vi "test2-DifferentChainNodesProcessDifferentAllowedMessages.vi"(8 "error in (no error)":errorcluster, 11 "TestCase in":refnum<class "testcase-CSMChainMode.lvclass">) -> (0 "error out":errorcluster, 3 "TestCase out":refnum<class "testcase-CSMChainMode.lvclass">)   [LabVIEW 2017, in "testcase-CSMChainMode.lvclass"]
uses:
  testcase-CSMChainMode.lvclass
  <vilib>/addons/_JKI Toolkits/VI Tester/TestCase.llb/TestCase.lvclass
  src/user.lib/_NEVSTOP/Communicable State Machine(CSM)/Communicable State Machine.lvlib
  C:/Program Files (x86)/National Instruments/LabVIEW 2017/vi.lib/addons/_JKI Toolkits/VI Tester/TestCase.llb/TestCase.lvclass
panel:
  out "LoopCount":i32
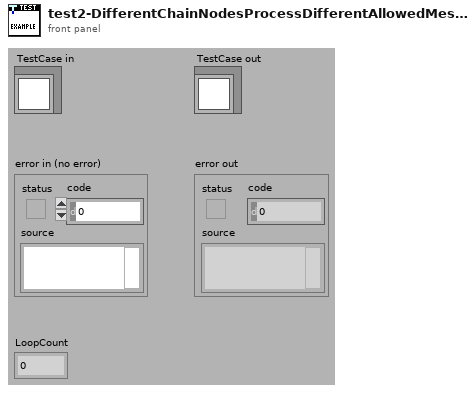
[diagram p1: front panel]
types:
  T1 = cluster{"Allowed":string, "Not Allowed":string[]}[]
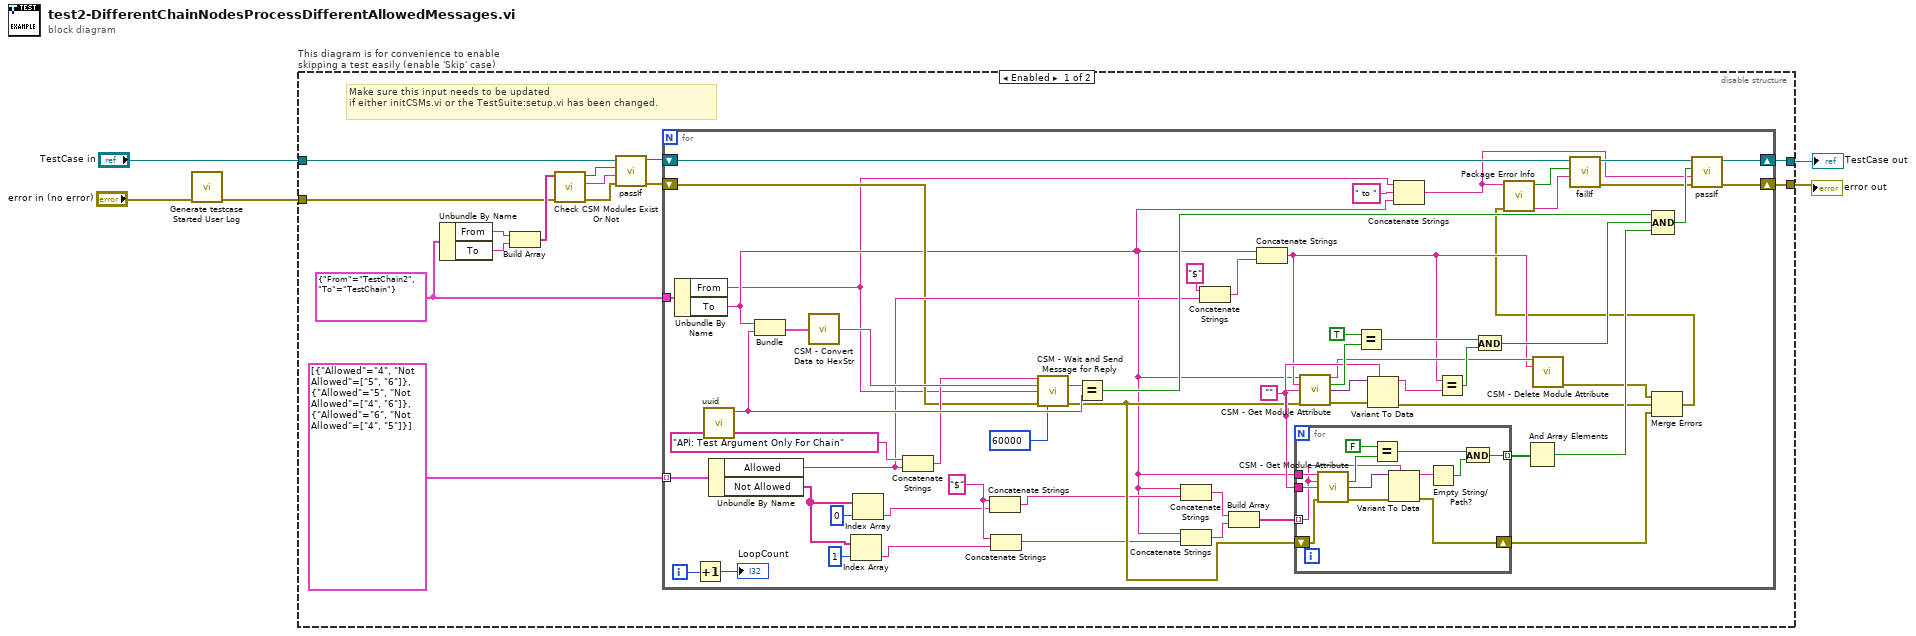
[diagram p0: block diagram]
diagram:
  n1 = call "Generate testcase Started User Log.vi"("Error In"="error in (no error)") -> ("error out"=w1:errorcluster)  [unwired: 10 in]
  n2 = disable-structure "This diagram is for convenience to enable skipping a test easily (enable 'Skip' case)" shown="Enabled" {
    disable-tunnel: "TestCase in" -> [w10 w93]
    disable-tunnel: [w19 w91] -> w2
    disable-tunnel: [w18 w92] -> w4
    disable-tunnel: w1 -> [w8 w90]
    frame Enabled {
      w6 = cluster{"From":string, "To":string} {"From"="TestChain2", "To"="TestChain"} ("Cluster")
      # "Make sure this input needs to be updated \nif either initCSMs.vi or the TestSuite:setup.vi has been changed."
      n3 = Unbundle By Name(w6) -> ("From"=w12:string, "To"=w13:string)
      n4 = Build Array(w12, w13) -> (w11:string[])
      n5 = call "Check CSM Modules Exist Or Not.vi"("error in"=w8, "CSM names in"=w11) -> ("error out"=w14:errorcluster, "Debug string"=w15:string, "All Modules Exist?"=w16:bool)  [unwired: 7 in]
      n6 = call-dynamic "passIf.vi"("error in (no error)"=w14, "message (\"\")"=w15, "pass"=w16, "TestCase in"=w10) -> ("error out"=w7:errorcluster, "TestCase out"=w9:refnum<class "testcase-CSMChainMode.lvclass">)  [unwired: 6 in]
      n7 = for {
        tunnel: w6 -> [w76]
        shift-right: [w71] -> w19
        shift-left: w9 -> [w27]
        shift-right: [w70] -> w18
        shift-left: w7 -> [w31]
        tunnel: T1 [{"Allowed"="4", "Not Allowed"=["5", "6"]}, {"Allowed"="5", "Not Allowed"=["4", "6"]}, {"Allowed"="6", "Not Allowed"=["4", "5"]}] -> [w48] mode=indexing
        i -> [w50]
        w42 = "$" ("string")
        w59 = ""
        n8 = Unbundle By Name(w76) -> ("From"=w22:string, "To"=w23:string)
        n9 = Increment(x=w50) -> (x+1=→"LoopCount":i32)
        n10 = call "uuid.vi"() -> ("UUID"=w62:string)  [unwired: 11 in]
        n11 = Unbundle By Name(w48) -> ("Allowed"=w44:string, "Not Allowed"=w38:string[])
        n12 = Bundle("To"=w23, "UUID"=w62) -> (w75:cluster{"To":string, "UUID":string})  [unwired: 1 in]
        n13 = call "CSM - Convert Data to HexStr.vi"("Variant"=w75) -> ("HEX String (0-9,A-F)"=w74:string)  [unwired: 8 in]
        n14 = Index Array(array=w38, index=1) -> (element=w37:string)
        n15 = Index Array(array=w38, index=0) -> (element=w40:string)
        n16 = Concatenate Strings("API: Test Argument Only For Chain" ("State"), w44) -> (w46:string)
        n17 = Concatenate Strings(w42, w40) -> (w36:string)
        n18 = Concatenate Strings(w42, w37) -> (w35:string)
        n19 = call "CSM - Wait and Send Message for Reply.vi"("State"=w46, "Arguments (\"\")"=w74, "Target Module"=w22, "Error In (No Error)"=w31, "Response Timeout (-2 Using Global Settings)"=60000) -> ("Response"=w63:string, "error out"=w53:errorcluster)  [unwired: 7 in, 2 out]
        n20 = Equal?(x=w63, y=w62) -> (x = y?=w73:bool)
        n21 = Concatenate Strings(w23, w36) -> (w58:string)
        n22 = Concatenate Strings(w23, w35) -> (w57:string)
        n23 = Concatenate Strings("$" ("string"), w44) -> (w43:string)
        n24 = Build Array(w58, w57) -> (w56:string[])
        n25 = Concatenate Strings(w23, w43) -> (w33:string)
        n26 = for {
          tunnel: w59 -> [w89]
          tunnel: w23 -> [w84]
          tunnel: w56 -> [w83] mode=indexing
          tunnel: [w79] -> w55 mode=indexing
          shift-right: [w77] -> w51
          shift-left: w53 -> [w78]
          n27 = call "CSM - Get Module Attribute.vi"("CSM Name"=w84, "Attribute"=w83, "Default Value (Empty Variant)"=w89, "Error In"=w78) -> ("Found"=w86:bool, "Value"=w87:variant, "error out"=w88:errorcluster)  [unwired: 7 in, 2 out]
          n28 = Equal?(x=FALSE, y=w86) -> (x = y?=w80:bool)
          n29 = Variant To Data(error in=w88, type=w83, Variant=w87) -> (data=w82:string, error out=w77:errorcluster)
          n30 = Empty String/Path?(string/path=w82) -> (empty?=w81:bool)
          n31 = And(x=w80, y=w81) -> (x .and. y?=w79:bool)
        }
        n32 = call "CSM - Get Module Attribute.vi"("CSM Name"=w23, "Attribute"=w33, "Default Value (Empty Variant)"=w59, "Error In"=w53) -> ("CSM Name (Dup)"=w34:string, "Found"=w69:bool, "Value"=w66:variant, "error out"=w67:errorcluster)  [unwired: 7 in, 1 out]
        n33 = Equal?(x=TRUE, y=w69) -> (x = y?=w65:bool)
        n34 = Variant To Data(error in=w67, type=w59, Variant=w66) -> (data=w61:string, error out=w52:errorcluster)
        n35 = Concatenate Strings(w22, " to " ("string"), w23) -> (w21:string)
        n36 = Equal?(x=w33, y=w61) -> (x = y?=w64:bool)
        n37 = And(x=w65, y=w64) -> (x .and. y?=w60:bool)
        n38 = And Array Elements(Boolean array=w55) -> (logical AND=w54:bool)
        n39 = call "CSM - Delete Module Attribute.vi"("CSM Name"=w34, "Attribute"=w33) -> ("error out"=w32:errorcluster)  [unwired: 10 in, 3 out]
        n40 = Compound Arithmetic op=AND(w73, w60, w54) -> (w72:bool)
        n41 = Merge Errors(w32, w52, w51) -> (w24:errorcluster)
        n42 = call "Package Error Info.vi"("error in"=w24, "String in"=w21) -> ("packed error info out"=w29:string, "error status"=w30:bool)  [unwired: 8 in]
        n43 = call-dynamic "failIf.vi"("message (\"\")"=w29, "fail"=w30, "TestCase in"=w27) -> ("error out"=w25:errorcluster, "TestCase out"=w26:refnum<class "testcase-CSMChainMode.lvclass">)  [unwired: 7 in]
        n44 = call-dynamic "passIf.vi"("error in (no error)"=w25, "message (\"\")"=w21, "pass"=w72, "TestCase in"=w26) -> ("error out"=w70:errorcluster, "TestCase out"=w71:refnum<class "testcase-CSMChainMode.lvclass">)  [unwired: 6 in]
      }
    }
    frame Disabled {
      # "skip test result while test is under development"
      n45 = call <vilib>:"skip.vi"("error in (no error)"=w90, "TestCase in"=w93) -> ("error out"=w92:errorcluster, "TestCase out"=w91:refnum<class "testcase-CSMChainMode.lvclass">)  [unwired: 8 in]
    }
  }
  "error out" <- w4
  "TestCase out" <- w2
